vi "Annotate Frame.vi"(8 "error in (no error)":errorcluster, 10 "Annotation":string, 11 "Frame Grabber Data In in":T1={"Camera Session"="", "Frame"=refnum, "AVI Refnum"=refnum, "Codecs"=[], "Frame number"=0, "Tracking File Refnum"=refnum, "Tick Count"=0, "Probe Object"=refnum, "Playback Probe Data"=[], "Rigid Body"={"Position"={"x (mm)"=0.0, "y (mm)"=0.0, "z (mm)"=0.0}, "Orientation"={"Pitch (rad)"=0.0, "Yaw (rad)"=0.0, "Roll (rad)"=0.0}, "Quaternion"={"qx"=0.0, "qy"=0.0, "qz"=0.0, "qw"=0.0}, "Tracked?"=FALSE}, "Total no frames playback"=0, "Video FPS"=0.0, "Camera connected?"=FALSE, "Scene"=refnum, "Cropped Frame"=refnum, "Tracker FPS"=0.0, "Crop ROI"=[], "Presentation Values"=[], "Elapsed time (ms)"=0, "Camera frames playback"=0, "Refnums"={"Live Refnum"=refnum, "Record Refnum"=refnum, "Recording Settings Refnum"=refnum, "Playback Refnum"=refnum, "Frame Slider Refnum"=refnum, "Pause Refnum"=refnum, "Home Refnum"=refnum, "Crop Refnum"=refnum, "Clear Crop Refnum"=refnum, "stop refnum"=refnum, "Playback Rate Refnum"=refnum, "Operator Settings Refnums"=refnum, "Presentation Refnum"=refnum, "Gestation Refnum"=refnum, "Crop Time Frame Slider Refnum"=refnum, "Cancel Save Refnum"=refnum, "Reverse Playback Refnum"=refnum, "Connection Settings Refnum"=refnum}, "Dimensions"={"Probe Dimensions"={"Probe Width"=0.0, "Probe Depth"=1.0, "Probe Height"=0.0}, "Room Dimensions"={"Room Width"=0.0, "Room Depth"=0.0, "Room Height"=0.0}}, "Playback Data As Strings"=[], "Cropped Tracking File Refnum"=refnum, "Cropped AVI Refnum"=refnum, "Header"=[], "Total euclidian distance"=0.0, "Annotation File Path"=path "", "Playback File Path"=path ""}) -> (0 "error out":errorcluster)   [LabVIEW 2017]
uses:
  Controls/Frame Grabber Data.ctl
  <vilib>/userdefined/High Color/IMAQdx.ctl
  <vilib>/vision/Image Controls.llb/IMAQ Image.ctl
  <vilib>/vision/Avi.llb/IMAQ AVI2 Refnum.ctl
  Controls/Rigid Body Info.ctl
  Controls/Position.ctl
  Controls/Orientation.ctl
  Controls/Refnums.ctl
  Controls/Recording Settings.ctl
  Controls/Operator Settings.ctl
  Controls/Operator.ctl
  Controls/Connection Settings.ctl
  Controls/Tracker Type.ctl
  Controls/COM Port.ctl
  Controls/Dimensions.ctl
  Controls/Room Dimensions.ctl
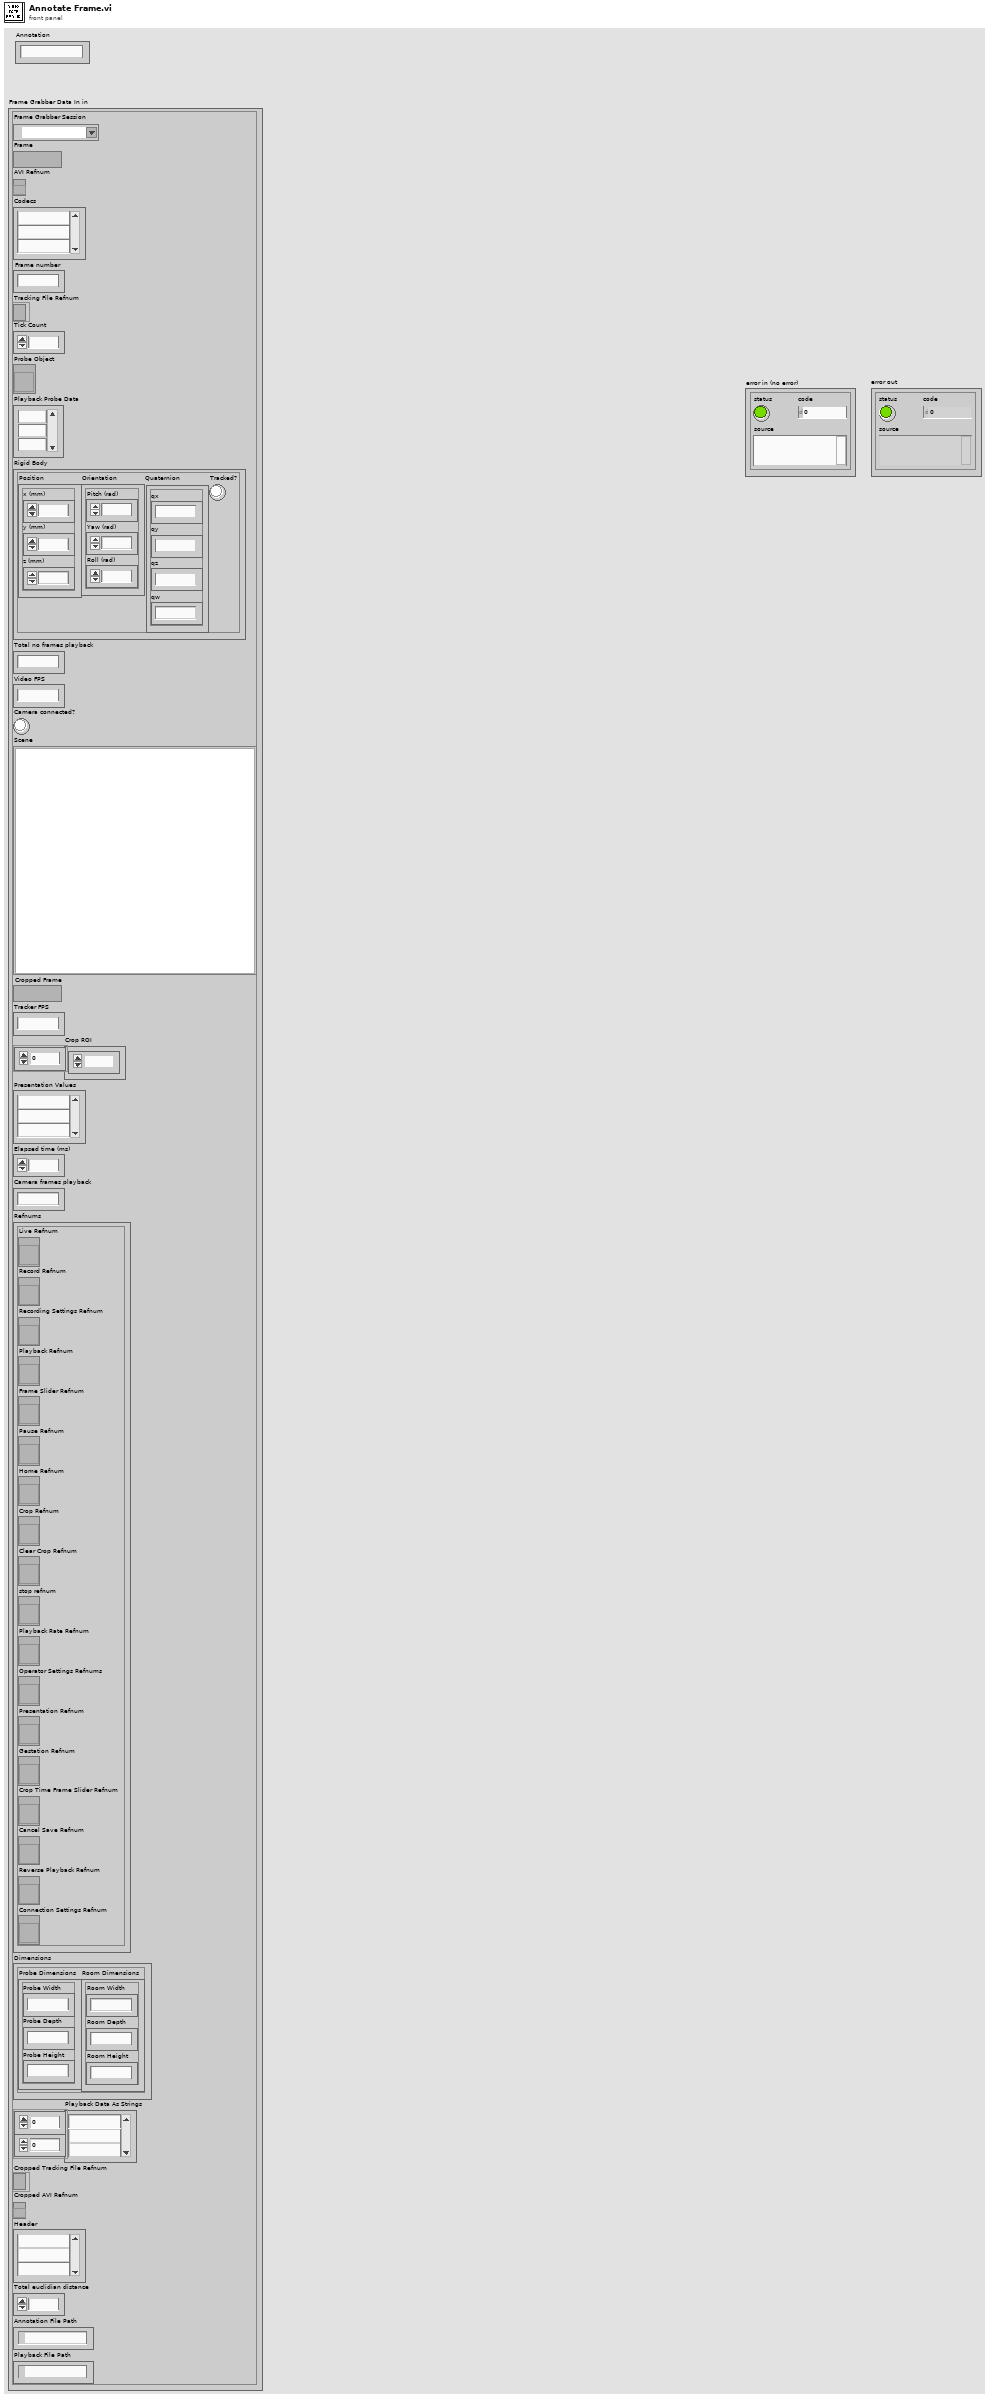
[diagram p1: front panel]
types:
  T1 = typedef "Frame Grabber Data.ctl" = cluster{"Camera Session":T2, "Frame":T3, "AVI Refnum":T4, "Codecs":string[], "Frame number":u32, "Tracking File Refnum":refnum<file>, "Tick Count":u32, "Probe Object":refnum<vi>, "Playback Probe Data":dbl[][], "Rigid Body":T5, "Total no frames playback":i32, "Video FPS":dbl, "Camera connected?":bool, "Scene":refnum<vi>, "Cropped Frame":T3, "Tracker FPS":dbl, "Crop ROI":i32[], "Presentation Values":string[], "Elapsed time (ms)":u32, "Camera frames playback":u32, "Refnums":T8, "Dimensions":T9, "Playback Data As Strings":string[][], "Cropped Tracking File Refnum":refnum<file>, "Cropped AVI Refnum":T4, "Header":string[], "Total euclidian distance":dbl, "Annotation File Path":path, "Playback File Path":path}
  T2 = typedef "IMAQdx.ctl" = refnum<k21>
  T3 = typedef "IMAQ Image.ctl" = refnum<image>
  T4 = typedef "IMAQ AVI2 Refnum.ctl" = refnum<k20>
  T5 = typedef "Rigid Body Info.ctl" = cluster{"Position":T6, "Orientation":T7, "Quaternion":cluster{"qx":sgl, "qy":sgl, "qz":sgl, "qw":sgl}, "Tracked?":bool}
  T6 = typedef "Position.ctl" = cluster{"x (mm)":sgl, "y (mm)":sgl, "z (mm)":sgl}
  T7 = typedef "Orientation.ctl" = cluster{"Pitch (rad)":sgl, "Yaw (rad)":sgl, "Roll (rad)":sgl}
  T8 = typedef "Refnums.ctl" = cluster{"Live Refnum":refnum<vi>, "Record Refnum":refnum<vi>, "Recording Settings Refnum":refnum<vi>, "Playback Refnum":refnum<vi>, "Frame Slider Refnum":refnum<vi>, "Pause Refnum":refnum<vi>, "Home Refnum":refnum<vi>, "Crop Refnum":refnum<vi>, "Clear Crop Refnum":refnum<vi>, "stop refnum":refnum<vi>, "Playback Rate Refnum":refnum<vi>, "Operator Settings Refnums":refnum<vi>, "Presentation Refnum":refnum<vi>, "Gestation Refnum":refnum<vi>, "Crop Time Frame Slider Refnum":refnum<vi>, "Cancel Save Refnum":refnum<vi>, "Reverse Playback Refnum":refnum<vi>, "Connection Settings Refnum":refnum<vi>}
  T9 = typedef "Dimensions.ctl" = cluster{"Probe Dimensions":cluster{"Probe Width":sgl, "Probe Depth":sgl, "Probe Height":sgl}, "Room Dimensions":T10}
  T10 = typedef "Room Dimensions.ctl" = cluster{"Room Width":dbl, "Room Depth":dbl, "Room Height":dbl}
  T11 = enum16{"open", "replace", "create", "open or create", "replace or create", "replace or create with confirmation"}
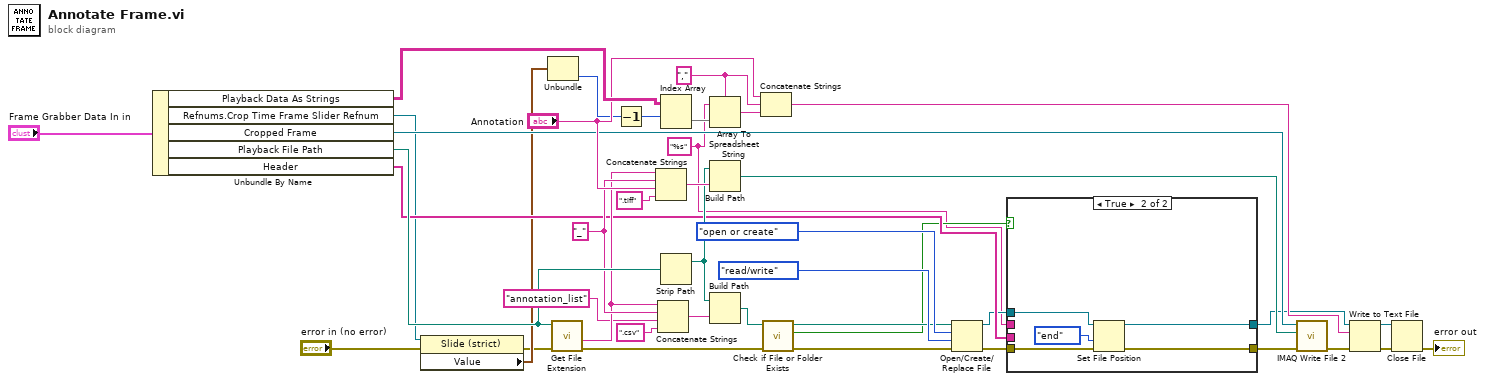
[diagram p0: block diagram]
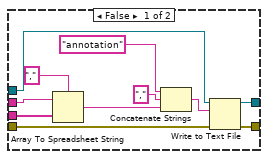
[diagram p2: hidden frame]
diagram:
  w24 = "_" ("string")
  w29 = "," ("delimiter (Tab)")
  w7 = "%s" ("format string")
  n1 = Unbundle By Name("Frame Grabber Data In in") -> ("Playback Data As Strings"=w40:string[][], "Refnums.Crop Time Frame Slider Refnum"=w6:refnum<vi>, "Cropped Frame"=w19:T3, "Playback File Path"=w38:path, "Header"=w14:string[])
  n2 = property class="Slide (strict)"(reference=w6, error in="error in (no error)") -> (error out=w2:errorcluster, "Value"=w5:cluster{i32, i32, i32})  [unwired: 1 out]
  n3 = Unbundle(w5) -> (w4:i32)  [unwired: 2 out]
  n4 = call <vilib>:"Get File Extension.vi"("error in (no error)"=w2, "file"=w38) -> ("error out"=w17:errorcluster, "filename without extension"=w23:string)  [unwired: 5 in, 3 out]
  n5 = Decrement(x=w4) -> (x-1=w1:i32)
  n6 = Concatenate Strings(w23, w24, "Annotation", ".tiff" ("string")) -> (w37:string)
  n7 = Concatenate Strings(w23, w24, "annotation_list" ("string"), ".csv" ("string")) -> (w34:string)
  n8 = Index Array(array=w40, index (row)=w1) -> (element=w8:string[])  [unwired: 1 in]
  n9 = Strip Path(path=w38) -> (stripped path=w33:path)  [unwired: 1 out]
  n10 = Array To Spreadsheet String(delimiter (Tab)=w29, array=w8, 3:w7) -> (spreadsheet string=w39:string)
  n11 = Build Path(base path=w33, name or relative path=w37) -> (appended path=w36:path)
  n12 = Build Path(base path=w33, name or relative path=w34) -> (appended path=w18:path)
  n13 = Concatenate Strings("Annotation", w29, w39) -> (w30:string)
  n14 = call <vilib>:"Check if File or Folder Exists.vi"("error in (no error)"=w17, "path"=w18) -> ("error out"=w16:errorcluster, "file or folder exists?"=w12:bool, "dup path"=w15:path)  [unwired: 7 in]
  n15 = Open/Create/Replace File(file path (use dialog)=w15, error in=w16, operation (0:open)=T11."open or create", access (0:read/write)=enum16{"read/write", "read-only", "write-only"}."read/write") -> (refnum out=w10:refnum<file>, error out=w13:errorcluster)  [unwired: 2 in, 1 out]
  n16 = case shown="True" w12 {
    tunnel: w14 -> [w45 _]
    tunnel: w13 -> [w50 w57]
    tunnel: [w49 w54] -> w11
    tunnel: w10 -> [w48 w56]
    tunnel: [w47 w55] -> w9
    tunnel: w7 -> [w42 _]
    frame False {
      n17 = Array To Spreadsheet String(delimiter (Tab)=",", array=w45, 3:w42) -> (spreadsheet string=w43:string)
      n18 = Concatenate Strings("annotation" ("string"), "," ("string"), w43) -> (w46:string)
      n19 = Write to Text File(file (use dialog)=w48, text=w46, error in=w50) -> (refnum out=w47:refnum<file>, error out=w49:errorcluster)  [unwired: 1 in, 1 out]
    }
    frame True {
      n20 = Set File Position(refnum=w56, from (0:start)=enum16{"start", "end", "current"}."end", error in=w57) -> (refnum out=w55:refnum<file>, error out=w54:errorcluster)  [unwired: 1 in]
    }
  }
  n21 = call-poly "IMAQ Write File 2"("error in (no error)"=w11, "File Path"=w36, "Image"=w19) -> ("error out"=w35:errorcluster)  [unwired: 7 in, 1 out]
  n22 = Write to Text File(file (use dialog)=w9, text=w30, error in=w35) -> (refnum out=w26:refnum<file>, error out=w27:errorcluster)  [unwired: 1 in, 1 out]
  n23 = Close File(refnum=w26, error in=w27) -> (error out=→"error out":errorcluster)  [unwired: 1 out]
